vi "Add to Mean.vi"(10 "Non Object":refnum<class "JSON Value.lvclass">, 11 "JSON Running Mean In":refnum<class "JSON Running Mean.lvclass">) -> (3 "JSON Running Mean":refnum<class "JSON Running Mean.lvclass">)   [LabVIEW 2020, in "Library Commun.lvlib" / "JSON Running Mean.lvclass"]
uses:
  JSON Running Mean.lvclass
  JSON Value/JSON Value.lvclass
  JSON Running Mean.lvclass/JSON Running Mean.ctl
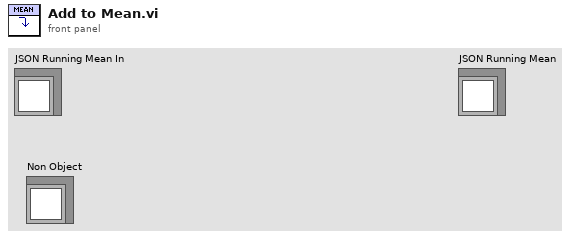
[diagram p1: front panel]
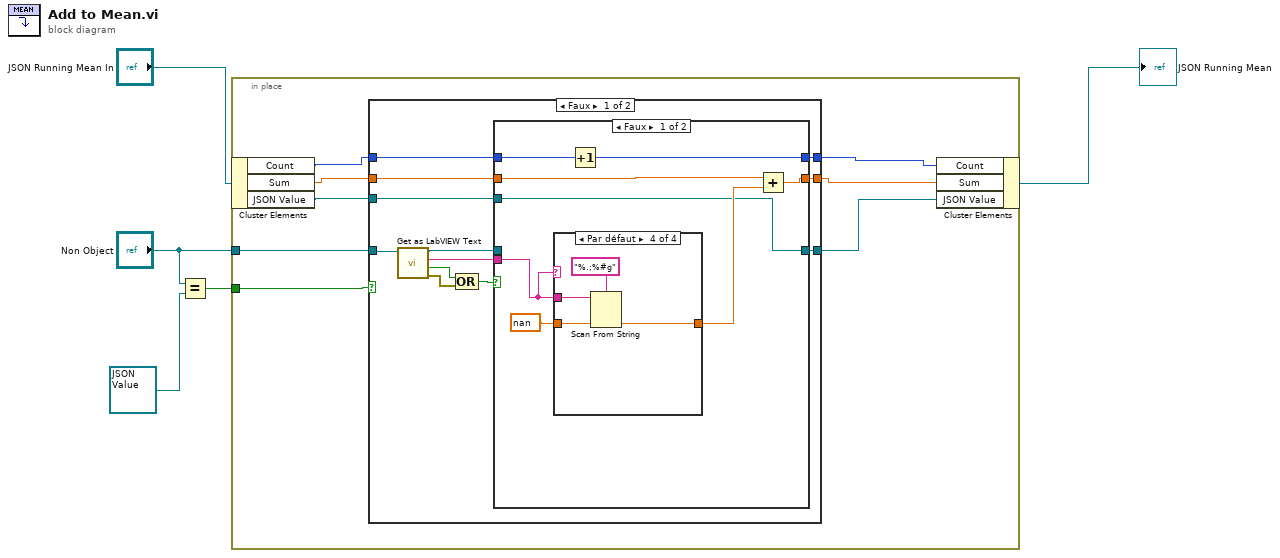
[diagram p0: block diagram]
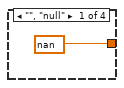
[diagram p2: hidden frame]
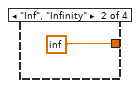
[diagram p3: hidden frame]
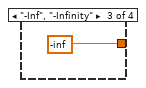
[diagram p4: hidden frame]
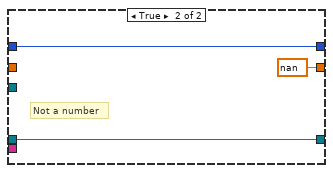
[diagram p5: hidden frame]
diagram:
  n1 = Equal?(x="Non Object", y=refnum<class "JSON Value.lvclass"> refnum) -> (x = y?=w4:bool)
  n2 = in-place {
    in-place-border: w4 -> [w13]
    in-place-border: "Non Object" -> [w12]
    n3 = in-place-cluster #1("JSON Running Mean In") -> ("Count"=w9:i32, "Sum"=w10:sgl, "JSON Value"=w11:refnum<class "JSON Value.lvclass">)
    n4 = case shown="Faux" w13 {
      tunnel: w10 -> [w25 w46]
      tunnel: [w24 w46] -> w7
      tunnel: w12 -> [w23 _]
      tunnel: [w15 w45] -> w6
      tunnel: w11 -> [w16 w45]
      tunnel: w9 -> [w18 w44]
      tunnel: [w17 w44] -> w8
      frame False {
        n5 = call-dynamic "Get as LabVIEW Text.vi"("JSON Value In"=w23) -> ("error out"=w20:errorcluster, "Was in quotes"=w21:bool, "LabVIEW Text"=w22:string, "JSON Value Out"=w14:refnum<class "JSON Value.lvclass">)  [unwired: 7 in]
        n6 = Compound Arithmetic op=OR(w21, w20) -> (w19:bool)
        n7 = case shown="Faux" w19 {
          tunnel: w25 -> [w33 _]
          tunnel: [w32 sgl nan] -> w24
          tunnel: w22 -> [w30 _]
          tunnel: w18 -> [w28 w43]
          tunnel: [w27 w43] -> w17
          tunnel: w16 -> [w26 _]
          tunnel: [w26 w41] -> w15
          tunnel: w14 -> [_ w41]
          frame False {
            n8 = case shown="Par défaut" w30 {
              tunnel: [sgl nan ("default value 1") sgl inf ("default value 1") sgl -inf ("default value 1") w38] -> w29
              tunnel: sgl nan ("default value 1") -> [_ _ _ w40]
              tunnel: w30 -> [_ _ _ w39]
              frame "", "null" {
              }
              frame "Inf", "Infinity" {
              }
              frame "-Inf", "-Infinity" {
              }
              frame Default {
                n9 = Scan From String(format string="%.;%#g", input string=w39, default 1=w40) -> (output 1=w38:sgl)  [unwired: 2 in, 3 out]
              }
            }
            n10 = Increment(x=w28) -> (x+1=w27:i32)
            n11 = Add(x=w33, y=w29) -> (x+y=w32:sgl)
          }
          frame True {
            # "Not a number"
          }
        }
      }
      frame True {
      }
    }
    n12 = in-place-cluster #1("Count"=w8, "Sum"=w7, "JSON Value"=w6) -> (→"JSON Running Mean":refnum<class "JSON Running Mean.lvclass">)
  }
